vi "Read Data.vi"(0 "comm interface in":refnum<class "RoboRIO UART.lvclass">, 5 "bytes to read":i32, 11 "error in":errorcluster) -> (4 "comm interface out":refnum<class "RoboRIO UART.lvclass">, 6 "data":u8[](array[numeric]), 15 "error out":errorcluster)   [LabVIEW 2018, in "RoboRIO UART.lvclass"]
uses:
  RoboRIO UART.lvclass
  RoboRIO UART.lvclass/RoboRIO UART.ctl
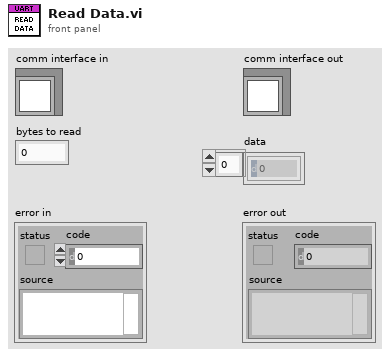
[diagram p1: front panel]
types:
  T1 = typedef "WPI_SerialPortRef.ctl" = cluster{"DevStatus":errorcluster, "Serial Port Name":refnum<visa-resource-name>}
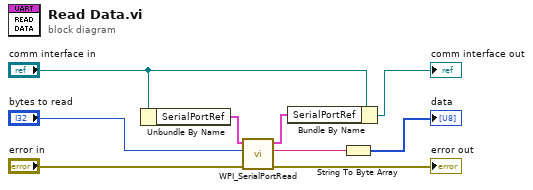
[diagram p0: block diagram]
diagram:
  n1 = Unbundle By Name("comm interface in") -> ("SerialPortRef"=w7:T1)
  n2 = call <vilib>:"WPI_SerialPortRead.vi"("error in (no error)"="error in", "Num Bytes to Read"="bytes to read", "SerialPortRef"=w7) -> ("error out"=→"error out":errorcluster, "Buffer"=w2:string, "SerialPortRef"=w6:T1)  [unwired: 6 in]
  n3 = Bundle By Name(cluster="comm interface in", "SerialPortRef"=w6) -> (→"comm interface out":refnum<class "RoboRIO UART.lvclass">)
  n4 = String To Byte Array(string=w2) -> (unsigned byte array=→"data":u8[])
